vi "getAPPDATA.vi"() -> (3 "APPDATA String/Binary data":string)   [LabVIEW 2013, in "Utilities.lvlib"]
uses:
  <vilib>/registry/registry.llb/Registry RtKey.ctl
  <vilib>/registry/registry.llb/Read Registry Value Simple STR.vi
  lib/Utilities.lvlib
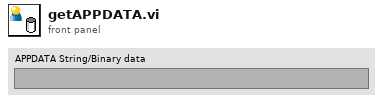
[diagram p1: front panel]
types:
  T1 = typedef "Registry RtKey.ctl" = enum32{"HKEY_CLASSES_ROOT", "HKEY_CURRENT_USER", "HKEY_LOCAL_MACHINE", "HKEY_USERS", "HKEY_PERFORMANCE_DATA", "HKEY_CURRENT_CONFIG", "HKEY_DYN_DATA"}
  T2 = typedef "Registry refnum.ctl" = refnum<k1>
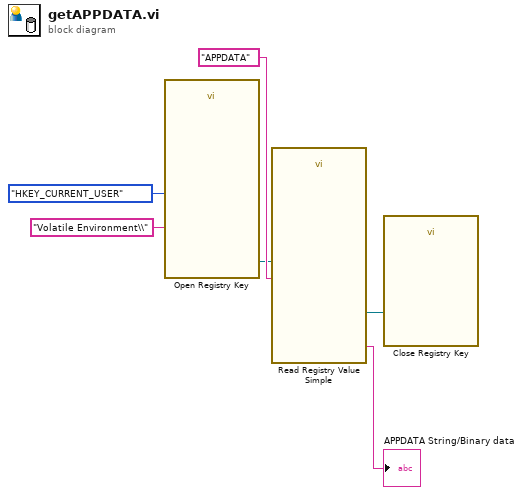
[diagram p0: block diagram]
diagram:
  n1 = call <vilib>:"Open Registry Key.vi"("subkey"="Volatile Environment\\", "root key (HKEY_LOCAL_MACHINE)"=Registry_RtKey."HKEY_CURRENT_USER") -> ("refnum out"=w1:T2)  [unwired: 8 in, 1 out]
  n2 = call-poly <vilib>:"Read Registry Value Simple.vi"("value"="APPDATA", "refnum"=w1) -> ("String/Binary data"=→"APPDATA String/Binary data":string, "refnum out"=w6:T2)  [unwired: 4 in, 2 out]
  n3 = call <vilib>:"Close Registry Key.vi"("refnum"=w6) -> ()  [unwired: 6 in, 1 out]
